vi "GetText.vi"(8 "error in":errorcluster, 11 "Fgen Channel in":refnum<class "Fgen Channel.lvclass">) -> (0 "error out":errorcluster, 1 "additional text":string, 2 "text":string, 3 "Fgen Channel out":refnum<class "Fgen Channel.lvclass">, 4 "glyph":string)   [LabVIEW 2025, in "Fgen.lvlib" / "Fgen Channel.lvclass"]
doc: "Copyright 2017 National Instruments Corporation\n\nLicensed under the Apache License, Version 2.0 (the \"License\"); you may not use this file except in compliance with the License. You may obtain a copy of the License at http://www.apache.org/licenses/LICENSE-2.0\nUnless required by applicable law or agreed to in writing, software distributed under the License is distributed on an \"AS IS\" BASIS, WITHOUT WARRANTIES OR CONDITIONS OF ANY KIND, either express or implied. See the License for the specific language governing permissions and limitations under the License."
uses:
  Fgen Channel.lvclass
  Fgen Channel.lvclass/Fgen Channel.ctl
  Fgen Channel configuration/Fgen Channel configuration.lvclass
  C:/Users/Public/Documents/Sandia National Labs/TSS Plugin/Abstract Engine.lvlibp/Plugin/Abstract/Channel configuration/Channel configuration.lvclass
  Users/Public/Documents/Sandia National Labs/TSS Plugin/Abstract Engine.lvlibp/Plugin/Abstract/Channel configuration/Read Channel Setting.vi
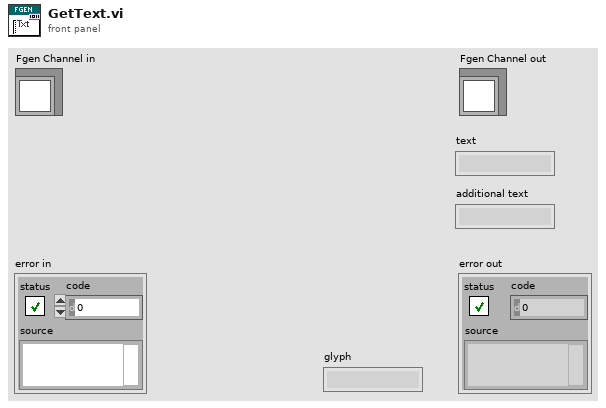
[diagram p1: front panel]
types:
  T1 = cluster{"Address":string, "SW Alias":string, "Description":string, "Enabled":bool, "Node Class":string}
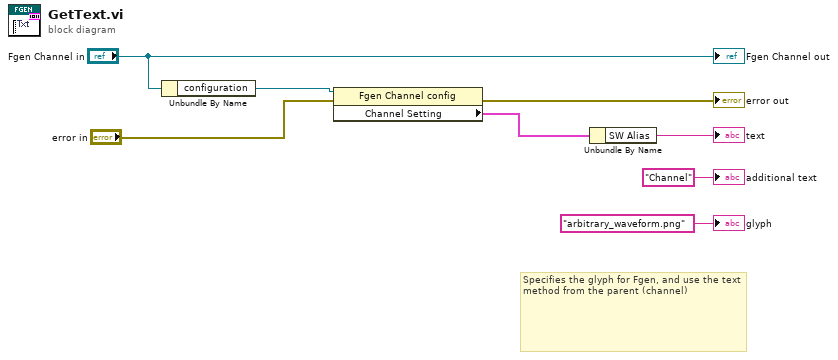
[diagram p0: block diagram]
diagram:
  # "Specifies the glyph for Fgen, and use the text method from the parent (channel)"
  n1 = Unbundle By Name("Fgen Channel in") -> ("configuration"=w6:refnum<class "Fgen Channel configuration.lvclass">)
  n2 = property class="Fgen Channel config"(reference=w6, error in="error in") -> (error out=→"error out":errorcluster, "Channel Setting"=w1:T1)  [unwired: 1 out]
  n3 = Unbundle By Name(w1) -> ("SW Alias"=→"text":string)
  "Fgen Channel out" <- "Fgen Channel in"
  "additional text" <- "Channel" ("additional text")
  "glyph" <- "arbitrary_waveform.png" ("glyph")
